vi "AngleCorrection.vi"(11 "Oiiginal":dbl[](array[numeric])) -> (3 "Modified":dbl[](array[numeric]))   [LabVIEW 2015]
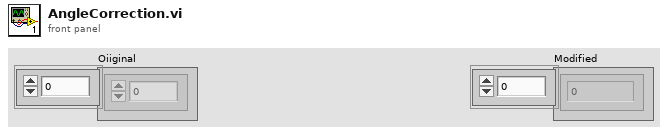
[diagram p1: front panel]
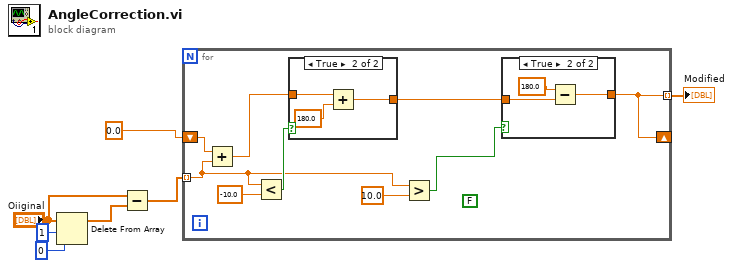
[diagram p0: block diagram]
diagram:
  n1 = Delete From Array(array="Oiiginal", length=1, index=0) -> (array with subset deleted=w2:dbl[])  [unwired: 1 out]
  n2 = Subtract(x="Oiiginal", y=w2) -> (x-y=w1:dbl[])
  n3 = for {
    tunnel: w1 -> [w9] mode=indexing
    shift-right: [w12] -> _
    shift-left: 0.0 -> [w15]
    tunnel: [w12] -> w6 mode=indexing
    (unwired) FALSE
    n4 = Add(x=w15, y=w9) -> (x+y=w14:dbl)
    n5 = Less?(x=w9, y=-10.0 ("x")) -> (x < y?=w16:bool)
    n6 = case shown="True" w16 {
      tunnel: w14 -> [w21 w23]
      tunnel: [w21 w22] -> w13
      frame False {
      }
      frame True {
        n7 = Add(x=w23, y=180.0) -> (x+y=w22:dbl)
      }
    }
    n8 = Greater?(x=w9, y=10.0 ("x")) -> (0:w8:bool)
    n9 = case shown="True" w8 {
      tunnel: [w17 w19] -> w12
      tunnel: w13 -> [w17 w18]
      frame False {
      }
      frame True {
        n10 = Subtract(x=180.0, y=w18) -> (x-y=w19:dbl)
      }
    }
  }
  "Modified" <- w6
